vi "Configure Power Measurement Parameter Set Mode.vi"(8 "error in (no error)":errorcluster, 9 "Parameter Set (Global)":i32(ring) items=["Global", "Independent"], 10 "Instance (1)":i32=1, 11 "VISA resource name":refnum<visa-resource-name>) -> (0 "error out":errorcluster, 3 "VISA resource name out":refnum<visa-resource-name>)   [LabVIEW 2020, in "Rohde&Schwarz CMXP GPRF.lvlib"]
doc: "Selects the measurement control settings for the power measurement.\n\nAttribute:\nRSCMXPGPRF_ATTR_POWER_MEASUREMENT_PARAMETER_SET_MODE\n\nRemote-control command:\nCONFigure:GPRF:MEAS<i>:POWer:PSET"
uses:
  <instrlib>/Rohde&Schwarz CMXP GPRF/Rohde&Schwarz CMXP GPRF.lvlib
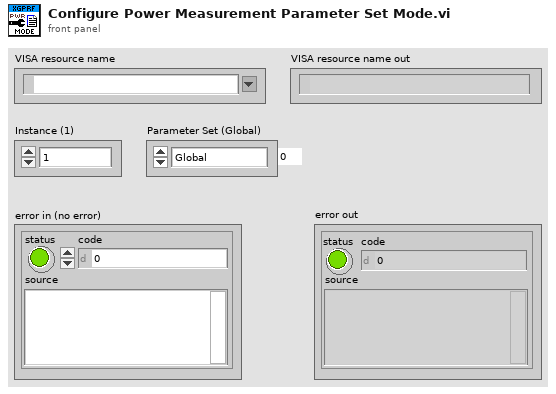
[diagram p1: front panel]
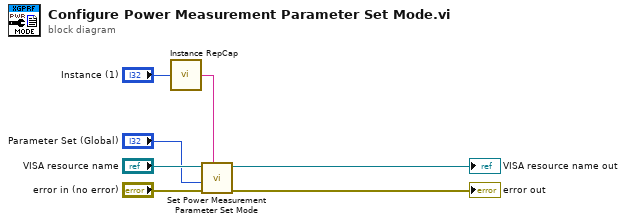
[diagram p0: block diagram]
diagram:
  n1 = call <instrlib>:"Instance RepCap.vi"("Instance in"="Instance (1)") -> ("Instance out"=w6:string)
  n2 = call "Set Power Measurement Parameter Set Mode"("Repeated Capabilities"=w6, "error in (no error)"="error in (no error)", "Power Measurement Parameter Set Mode (0 - Global)"="Parameter Set (Global)", "instrument handle"="VISA resource name") -> ("error out"=→"error out":errorcluster, "instrument handle out"=→"VISA resource name out":refnum<visa-resource-name>)  [unwired: 6 in]
